vi "Write_parameter.vi"(8 "error in (no error)":errorcluster caption="entrée d'erreur (pas d'erreur)", 10 "Parameter":string, 11 "Class Instrument (Default) en entrée":refnum<class "Class Instrument (Default).lvclass">) -> (0 "error out":errorcluster caption="sortie d'erreur", 3 "Class Instrument (Default) en sortie":refnum<class "Class Instrument (Default).lvclass">)   [LabVIEW 2020, in "Library Instrument & Equipement.lvlib" / "Library Instruments.lvlib" / "Class Instrument (Default).lvclass"]
uses:
  Class Instrument (Default).lvclass
  Class Instrument (Default).lvclass/Class Instrument (Default).ctl
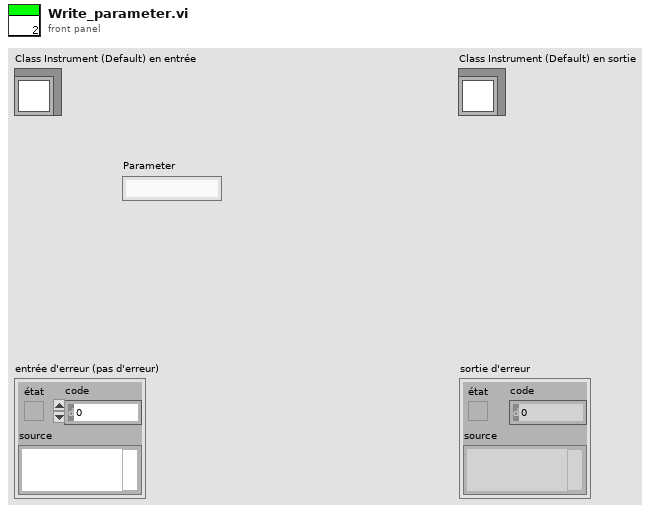
[diagram p1: front panel]
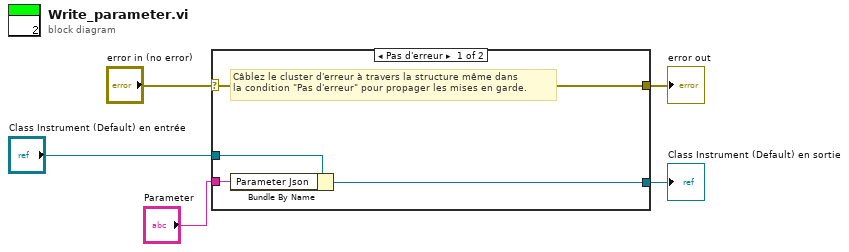
[diagram p0: block diagram]
diagram:
  n1 = case shown="Pas d'erreur" "error in (no error)" {
    selector: "error in (no error)" -> [w9 w11]
    tunnel: [w9 w11] -> w4
    tunnel: [w7 w10] -> w2
    tunnel: "Class Instrument (Default) en entrée" -> [w8 w10]
    tunnel: "Parameter" -> [w6 _]
    frame No Error {
      # "Câblez le cluster d'erreur à travers la structure même dans\nla condition \"Pas d'erreur\" pour propager les mises en garde."
      n2 = Bundle By Name(cluster=w8, "Parameter Json"=w6) -> (w7:refnum<class "Class Instrument (Default).lvclass">)
    }
    frame Error {
    }
  }
  "error out" <- w4
  "Class Instrument (Default) en sortie" <- w2
